vi "CRYASIOLaunchControlPanel.vi"(9 "Fs":i32=44100, 10 "Driver Name":string, 11 "error in (no error)":errorcluster) -> (3 "error out":errorcluster)   [LabVIEW 2013]
uses:
  CRY_ASIO.dll
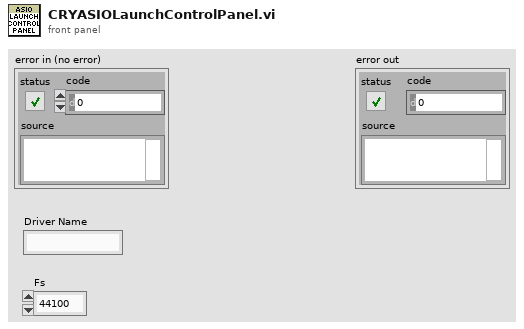
[diagram p1: front panel]
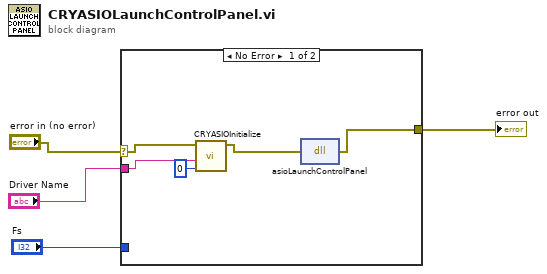
[diagram p0: block diagram]
diagram:
  n1 = case shown="No Error" "error in (no error)" {
    selector: "error in (no error)" -> [w8 w10]
    tunnel: [w9 w10] -> w3
    tunnel: "Driver Name" -> [w6 _]
    tunnel: "Fs" -> [_ _]
    frame No Error {
      n2 = call "CRYASIOInitialize.vi"("Sampling Rate"=u32 0, "Driver Name"=w6, "error in (no error)"=w8) -> ("error out"=w7:errorcluster)  [unwired: 7 in, 1 out]
      n3 = dll-call lib="D:/LabView_Project/CRY6181/CRY_ASIO.dll" fn="asioLaunchControlPanel"(error in=w7) -> (error out=w9:errorcluster)  [unwired: 3 in, 1 out]
    }
    frame Error {
    }
  }
  "error out" <- w3
